vi "Write Single Coil.vi"(8 "error in":errorcluster, 9 "coil to write":bool, 10 "address":u16, 11 "Modbus master in":refnum<class "Modbus Master.lvclass">) -> (0 "error out":errorcluster, 3 "Modbus master out":refnum<class "Modbus Master.lvclass">)   [LabVIEW 2014, in "MyLib.lvlib" / "Modbus Master.lvclass"]
doc: "Writes <B>coil to write</B> to <B>address</B> of the device."
uses:
  Modbus Master.lvclass
  Modbus Master.lvclass/Modbus Master.ctl
  Modbus API.lvclass/Modbus API.ctl
  Transmission Data Unit/Transmission Data Unit.lvclass
  Master Function Definition/Master Function Definition.lvclass
  Modbus API.lvclass
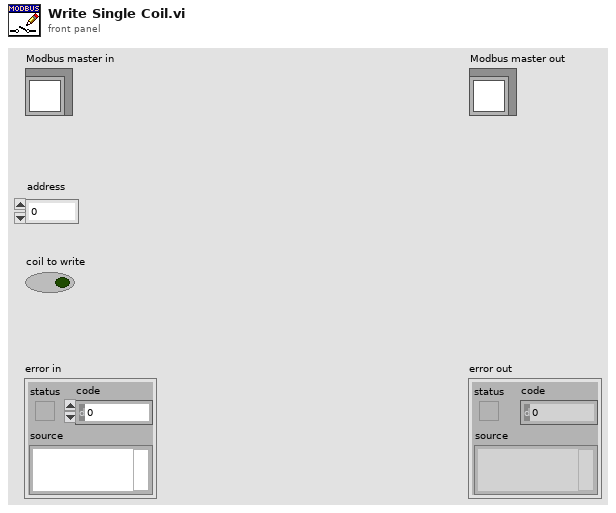
[diagram p1: front panel]
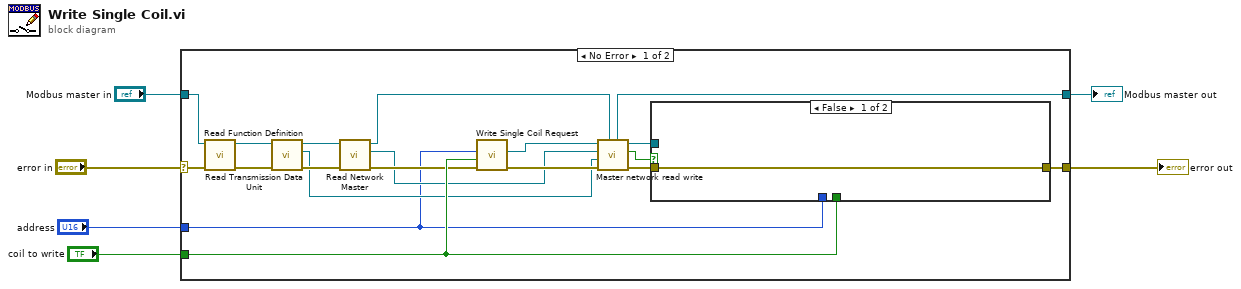
[diagram p0: block diagram]
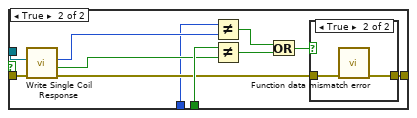
[diagram p2: hidden frame]
diagram:
  n1 = case shown="No Error" "error in" {
    selector: "error in" -> [w14 w42]
    tunnel: "Modbus master in" -> [w13 w41]
    tunnel: [w24 w42] -> w3
    tunnel: [w19 w41] -> w2
    tunnel: "address" -> [w8 _]
    tunnel: "coil to write" -> [w23 _]
    frame No Error {
      n2 = call "Read Function Definition.vi"("error in"=w14, "Modbus master in"=w13) -> ("error out"=w17:errorcluster, "Modbus master out"=w16:refnum<class "Modbus Master.lvclass">)  [unwired: 7 in, 1 out]
      n3 = call "Read Transmission Data Unit.vi"("error in"=w17, "Modbus instance in"=w16) -> ("error out"=w15:errorcluster, "transmission data unit"=w9:refnum<class "Transmission Data Unit.lvclass">, "Modbus instance out"=w18:refnum<class "Modbus Master.lvclass">)  [unwired: 7 in]
      n4 = call "Read Network Master.vi"("error in"=w15, "Modbus master in"=w18) -> ("error out"=w12:errorcluster, "network master"=w10:refnum<class "Network Master.lvclass">, "Modbus master out"=w11:refnum<class "Modbus Master.lvclass">)  [unwired: 7 in]
      n5 = call "Write Single Coil Request.vi"("error in"=w12, "Coil Value"=w23, "Starting Address"=w8) -> ("error out"=w25:errorcluster, "modbus data unit out"=w21:refnum<class "Modbus Data Unit.lvclass">)  [unwired: 7 in]
      n6 = call "Master network read write.vi"("Modbus master in"=w11, "error in"=w25, "transmission data unit in"=w9, "network master in"=w10, "Modbus data unit in"=w21) -> ("error out"=w22:errorcluster, "PDU Valid?"=w7:bool, "Modbus data unit out"=w20:refnum<class "Modbus Data Unit.lvclass">, "Modbus master out"=w19:refnum<class "Modbus Master.lvclass">)  [unwired: 3 in]
      n7 = case shown="False" w7 {
        tunnel: [w26 w36] -> w24
        tunnel: w23 -> [_ w32]
        tunnel: w22 -> [w26 w30]
        tunnel: w20 -> [_ w29]
        tunnel: w8 -> [_ w27]
        frame False {
        }
        frame True {
          n8 = call "Write Single Coil Response.vi"("error in"=w30, "modbus data unit in"=w29) -> ("error out"=w28:errorcluster, "Coil Value"=w31:bool, "Address"=w33:u16)  [unwired: 7 in]
          n9 = Not Equal?(x=w27, y=w33) -> (x != y?=w35:bool)
          n10 = Not Equal?(x=w32, y=w31) -> (x != y?=w34:bool)
          n11 = Or(x=w35, y=w34) -> (x .or. y?=w37:bool)
          n12 = case shown="True" w37 {
            tunnel: [w38 w40] -> w36
            tunnel: w28 -> [w38 w39]
            frame False {
            }
            frame True {
              n13 = call "Function data mismatch error.vi"("error in (no error)"=w39) -> ("error out"=w40:errorcluster)  [unwired: 10 in]
            }
          }
        }
      }
    }
    frame Error {
    }
  }
  "error out" <- w3
  "Modbus master out" <- w2
